vi "MapPositionSend.vi"(8 "error in (no error)":errorcluster caption="错误输入（无错误）", 10 "MapPosition":T1, 11 "States.lvlib:Guide.lvclass":refnum<class "Guide.lvclass">) -> (0 "error out":errorcluster caption="错误输出", 3 "Process State out":refnum<class "State Actor.lvclass">)   [LabVIEW 2014, in "States.lvlib" / "Guide.lvclass"]
uses:
  Guide.lvclass
  <vilib>/NI/Actors/State Actor/State Actor/State Actor.lvclass
  <vilib>/ActorFramework/Message Enqueuer/Message Enqueuer.lvclass/Message Enqueuer.ctl
  <vilib>/ActorFramework/Message Enqueuer/Enqueue.vi
  Global_var/Global_var.vi
  <vilib>/ActorFramework/Message Priority Queue/Priority Enqueue.vi
  Dialogue_lib/DialogueActor/Dialogue.lvclass
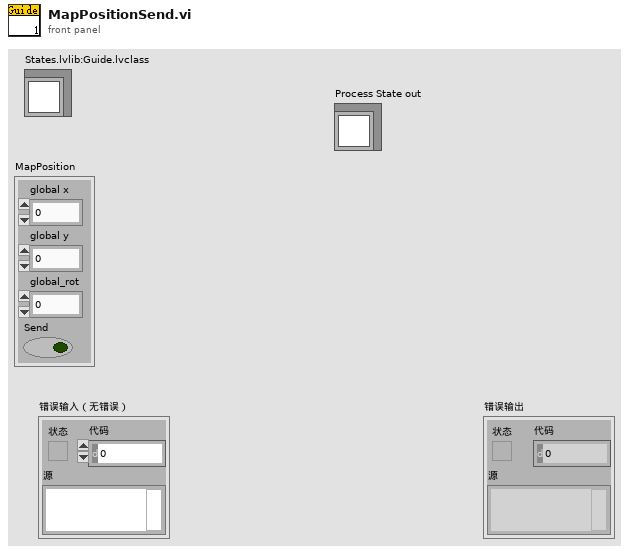
[diagram p1: front panel]
types:
  T1 = cluster{"global x":dbl, "global y":dbl, "global_rot":dbl, "Send":bool}
  T2 = cluster{"now_pose_X":dbl, "now_pose_Y":dbl, "now_pose_Rot_deg":dbl}
  T3 = cluster{"pose_X":dbl, "pose_Y":dbl, "pose_z":dbl, "pose_rot":dbl, "force_bool":bool}[]
  T4 = cluster{"pose_X":dbl, "pose_Y":dbl, "pose_z":dbl, "pose_rot":dbl, "force_bool":bool}
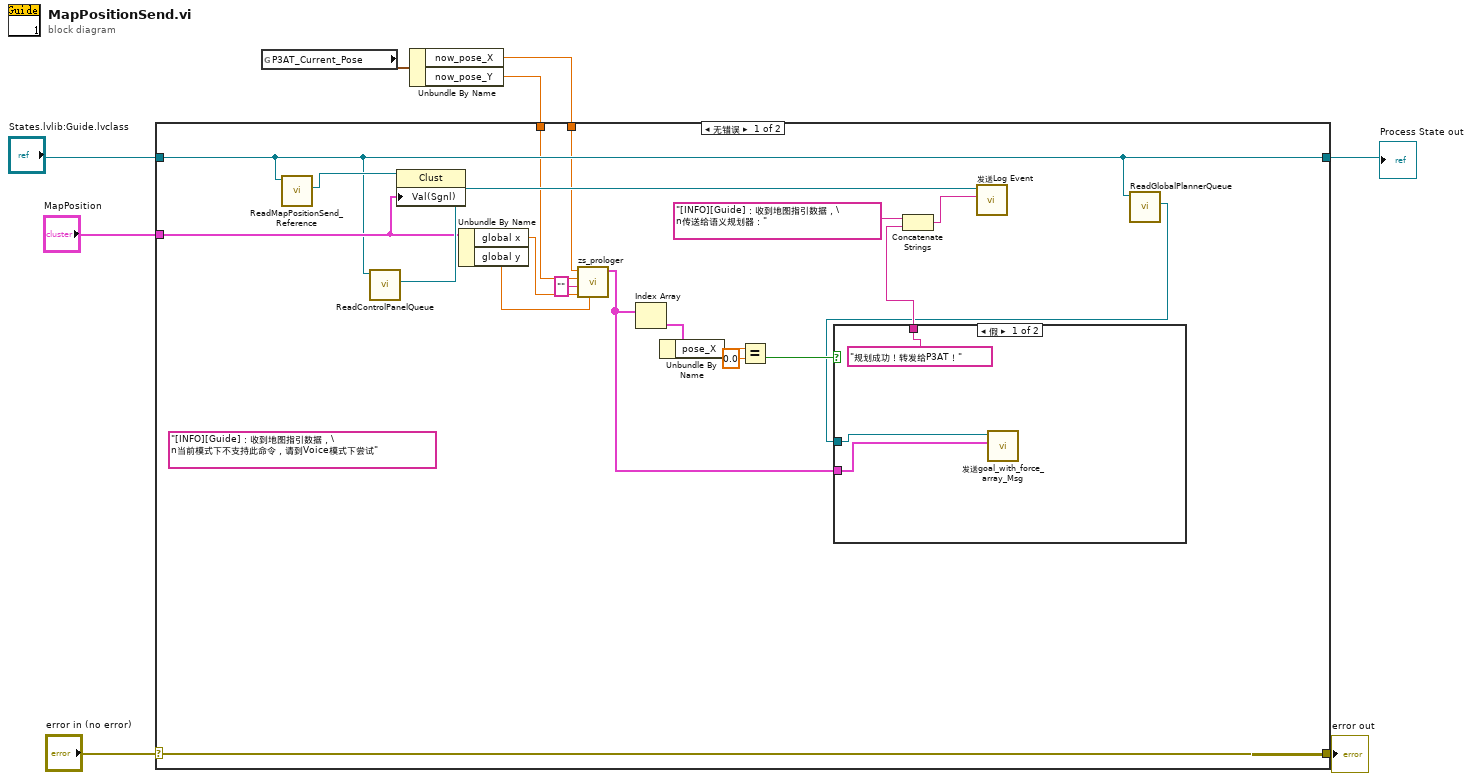
[diagram p0: block diagram]
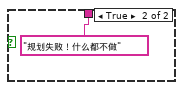
[diagram p2: hidden frame]
diagram:
  n1 = global read "Global_var.vi" "P3AT_Current_Pose"() -> (w3:T2)
  n2 = Unbundle By Name(w3) -> ("now_pose_X"=w2:dbl, "now_pose_Y"=w1:dbl)
  n3 = case shown="无错误" "error in (no error)" {
    selector: "error in (no error)" -> [w27 w32]
    tunnel: [w27 w32] -> w7
    tunnel: [w16 w33] -> w5
    tunnel: "States.lvlib:Guide.lvclass" -> [w16 w33]
    tunnel: "MapPosition" -> [w24 _]
    tunnel: w2 -> [w13 _]
    tunnel: w1 -> [w12 _]
    frame No Error {
      (unwired) "[INFO][Guide]：收到地图指引数据，\n当前模式下不支持此命令，请到Voice模式下尝试" ("Event Text")
      n4 = call-dynamic "ReadMapPositionSend_Reference.vi"("CoordinatorState输入"=w16) -> ("MapPositionSend_Reference"=w25:refnum<vi>)  [unwired: 8 in, 2 out]
      n5 = call-dynamic "ReadControlPanelQueue.vi"("CoordinatorState输入"=w16) -> ("操作者框架:消息待入队列"=w26:refnum<class "Message Enqueuer.lvclass">)  [unwired: 8 in, 2 out]
      n6 = property class="Clust"(reference=w25, "Val(Sgnl)"=w24) -> ()  [unwired: 1 in, 2 out]
      n7 = Unbundle By Name(w24) -> ("global x"=w11:dbl, "global y"=w10:dbl)
      n8 = call "zs_prologer.vi"("goal_y"=w10, "goal_x"=w11, "goal_node"="", "y"=w12, "x"=w13) -> ("goal_array"=w14:T3)  [unwired: 4 in]
      n9 = Index Array(array=w14) -> (element=w23:T4)  [unwired: 1 in]
      n10 = Unbundle By Name(w23) -> ("pose_X"=w22:dbl)
      n11 = Equal?(x=w22, y=0.0) -> (x = y?=w20:bool)
      n12 = call-dynamic "ReadGlobalPlannerQueue.vi"("CoordinatorState输入"=w16) -> ("操作者框架:消息待入队列"=w15:refnum<class "Message Enqueuer.lvclass">)  [unwired: 8 in, 2 out]
      n13 = case shown="假" w20 {
        tunnel: ["规划成功！转发给P3AT！" "规划失败！什么都不做"] -> w18
        tunnel: w15 -> [w29 _]
        tunnel: w14 -> [w28 _]
        frame False {
          n14 = call "发送goal_with_force_array_Msg.vi"("值(信号)"=w28, "消息待入队列"=w29) -> ()  [unwired: 8 in, 2 out]
        }
        frame True {
        }
      }
      n15 = Concatenate Strings("[INFO][Guide]：收到地图指引数据，\n传送给语义规划器：" ("Event Text"), w18) -> (w17:string)
      n16 = call "发送Log Event.vi"("Event Text"=w17, "消息待入队列"=w26) -> ()  [unwired: 8 in, 2 out]
    }
    frame Error {
    }
  }
  "error out" <- w7
  "Process State out" <- w5
